vi "DAC_lock_in_init.vi"(1 "Inst info":T1, 2 "FPGA VI Reference In":T2) -> ()   [LabVIEW 2013]
uses:
  fpga-bitfile-ref.ctl
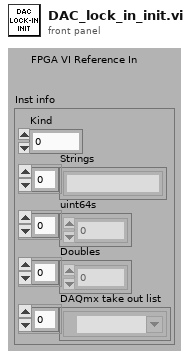
[diagram p1: front panel]
types:
  T1 = cluster{"Kind":u16, "Strings":string[], "uint64s":u64[], "Doubles":dbl[], "DAQmx take out list":refnum<k21>[]}
  T2 = typedef "fpga-bitfile-ref.ctl" = refnum<k20>
  T3 = enum16{"frequency", "channel", "amplitude", "inhibate"}
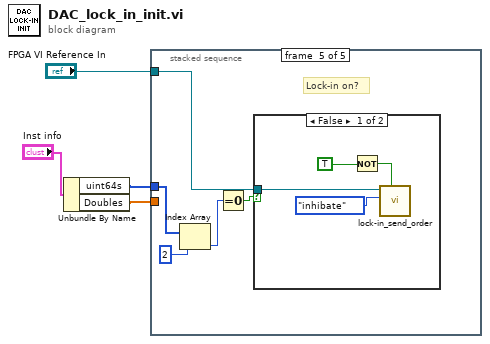
[diagram p0: block diagram]
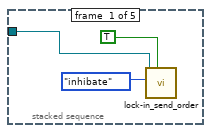
[diagram p2: hidden frame]
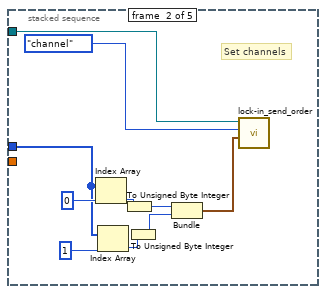
[diagram p3: hidden frame]
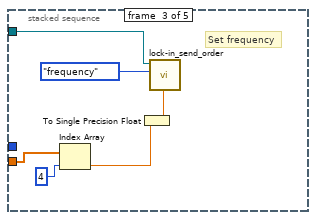
[diagram p4: hidden frame]
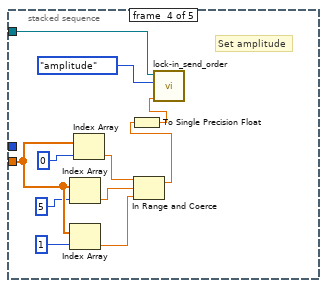
[diagram p5: hidden frame]
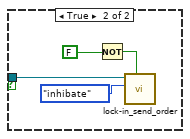
[diagram p6: hidden frame]
diagram:
  n1 = Unbundle By Name("Inst info") -> ("uint64s"=w2:u64[], "Doubles"=w1:dbl[])
  n2 = stacked-sequence {
    tunnel: "FPGA VI Reference In" -> [w7 w17 w22 w33 w35]
    tunnel: w2 -> [_ w8 _ _ w39]
    tunnel: w1 -> [_ _ w21 w32 _]
    frame #0 {
      n3 = call "lock-in_send_order.vi"("inhibate?"=TRUE, "order"=T3."inhibate", "FPGA VI Reference In"=w7) -> ()  [unwired: 4 in, 5 out]
    }
    frame #1 {
      # "Set channels"
      n4 = Index Array(array=w8, index=0) -> (element=w13:u64)
      n5 = Index Array(array=w8, index=1) -> (element=w12:u64)
      n6 = To Unsigned Byte Integer(number=w13) -> (unsigned 8bit integer=w10:u8)
      n7 = To Unsigned Byte Integer(number=w12) -> (unsigned 8bit integer=w9:u8)
      n8 = Bundle(w10, w9) -> (w11:cluster{u8, u8})  [unwired: 1 in]
      n9 = call "lock-in_send_order.vi"("Chanel (cl)"=w11, "order"=T3."channel", "FPGA VI Reference In"=w17) -> ()  [unwired: 3 in, 6 out]
    }
    frame #2 {
      # "Set frequency"
      n10 = Index Array(array=w21, index=4) -> (element=w19:dbl)
      n11 = To Single Precision Float(number=w19) -> (single precision float=w18:sgl)
      n12 = call "lock-in_send_order.vi"("frequency (Hz)"=w18, "order"=T3."frequency", "FPGA VI Reference In"=w22) -> ()  [unwired: 3 in, 6 out]
    }
    frame #3 {
      # "Set amplitude"
      n13 = Index Array(array=w32, index=5) -> (element=w30:dbl)
      n14 = Index Array(array=w32, index=1) -> (element=w29:dbl)
      n15 = Index Array(array=w32, index=0) -> (element=w31:dbl)
      n16 = In Range and Coerce(upper limit=w31, x=w30, lower limit=w29) -> (coerced(x)=w28:dbl)  [unwired: 1 out]
      n17 = To Single Precision Float(number=w28) -> (single precision float=w27:sgl)
      n18 = call "lock-in_send_order.vi"("amplitude"=w27, "order"=T3."amplitude", "FPGA VI Reference In"=w33) -> ()  [unwired: 3 in, 6 out]
    }
    frame #4 {
      # "Lock-in on?"
      n19 = Index Array(array=w39, index=2) -> (element=w36:u64)
      n20 = Equal To 0?(x=w36) -> (x = 0?=w37:bool)
      n21 = case shown="False" w37 {
        tunnel: w35 -> [w40 w46]
        frame False {
          n22 = Not(x=TRUE) -> (.not. x?=w42:bool)
          n23 = call "lock-in_send_order.vi"("inhibate?"=w42, "order"=T3."inhibate", "FPGA VI Reference In"=w40) -> ()  [unwired: 4 in, 5 out]
        }
        frame True {
          n24 = Not(x=FALSE) -> (.not. x?=w45:bool)
          n25 = call "lock-in_send_order.vi"("inhibate?"=w45, "order"=T3."inhibate", "FPGA VI Reference In"=w46) -> ()  [unwired: 4 in, 5 out]
        }
      }
    }
  }
